vi "array -- find index - real.vi"(8 "number":dbl, 11 "temperatures":dbl[](array[numeric])=[10.0, 20.0, 56.0, 92.0, 120.0, 183.0, 194.0, 310.0]) -> (0 "selector":T1, 1 "left index":i32, 2 "closest element index":i32, 3 "exact match ?":bool)   [LabVIEW 2015]
uses:
  comparison control.ctl
  Q - not nan -- real.vi
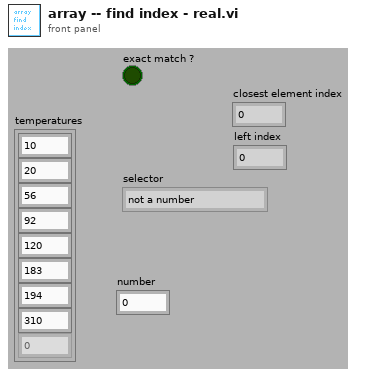
[diagram p1: front panel]
types:
  T1 = typedef "comparison control.ctl" = enum16{"not a number", "above", "in range", "below"}
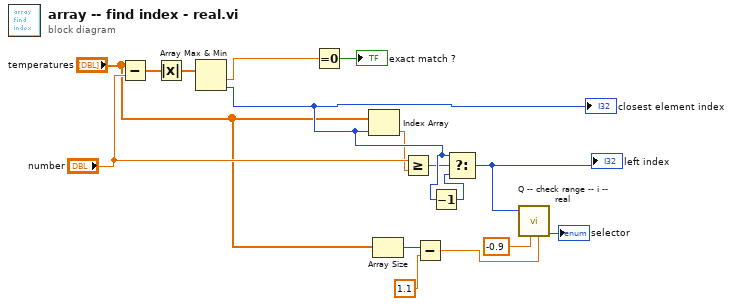
[diagram p0: block diagram]
diagram:
  n1 = Subtract(x="temperatures", y="number") -> (x-y=w16:dbl[])
  n2 = Absolute Value(x=w16) -> (abs(x)=w15:dbl[])
  n3 = Array Max & Min(array=w15) -> (min value=w2:dbl, min index (indices)=w14:i32)  [unwired: 2 out]
  "closest element index" <- w14
  n4 = Equal To 0?(x=w2) -> (x = 0?=→"exact match ?":bool)
  n5 = Index Array(array="temperatures", index=w14) -> (element=w12:dbl)
  n6 = Array Size(array="temperatures") -> (size(s)=w5:i32)
  n7 = Greater Or Equal?(x="number", y=w12) -> (x >= y?=w11:bool)
  n8 = Subtract(x=w5, y=1.1) -> (x-y=w3:dbl)
  n9 = Decrement(x=w14) -> (x-1=w10:i32)
  n10 = Select(t=w14, s=w11, f=w10) -> (s? t:f=w9:i32)
  "left index" <- w9
  n11 = call "Q -- check range -- i -- real.vi"("upper"=w3, "lower"=-0.9, "number"=w9) -> ("selector"=→"selector":T1)  [unwired: 6 in, 2 out]
